vi "Insert Bundle Unbundle.vi"(8 "error in (no error)":errorcluster, 10 "Diagnostic VI Path":string, 11 "QD Launch VI Ref":refnum<vi>) -> (0 "error out":errorcluster, 3 "changes made?":bool)   [LabVIEW 2017]
doc: "把选中的多条 wire 按自上而下的位置顺序 Bundle 成一个 cluster，再 Unbundle 后接回原来的源端子与下游端子，数据流保持不变。\n\n限制：每根选中的 wire 只能有一个下游端子（无分叉）；有分叉时报错并放弃，不改动框图。\n\n输入：\nQD Launch VI Ref - QuickDrop 启动所在的 VI，取其 Block Diagram 的 Selection List[]（正常使用方式）。\nDiagnostic VI Path - 非空时改为打开该路径的 VI 并对该框图内所有 wire 操作，结束时保存该 VI（测试/批处理用）。\n\n输出：\nerror out - 选中对象不全是 wire、少于 2 根、或存在分叉时返回错误。\nchanges made? - 是否实际改动了框图。\n\nUndo 事务由调用方（QuickDrop 插件模板）管理。"
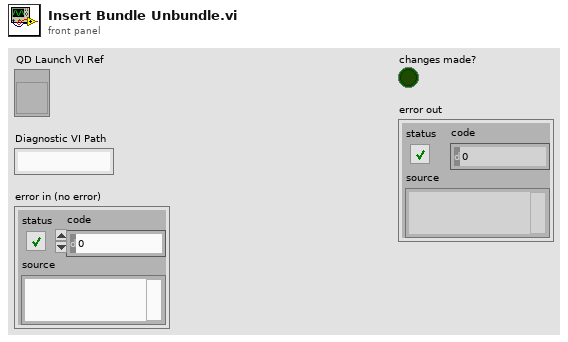
[diagram p1: front panel]
types:
  T1 = typedef "LVRectTypeDef.ctl" = cluster{"Left":i16, "Top":i16, "Right":i16, "Bottom":i16}
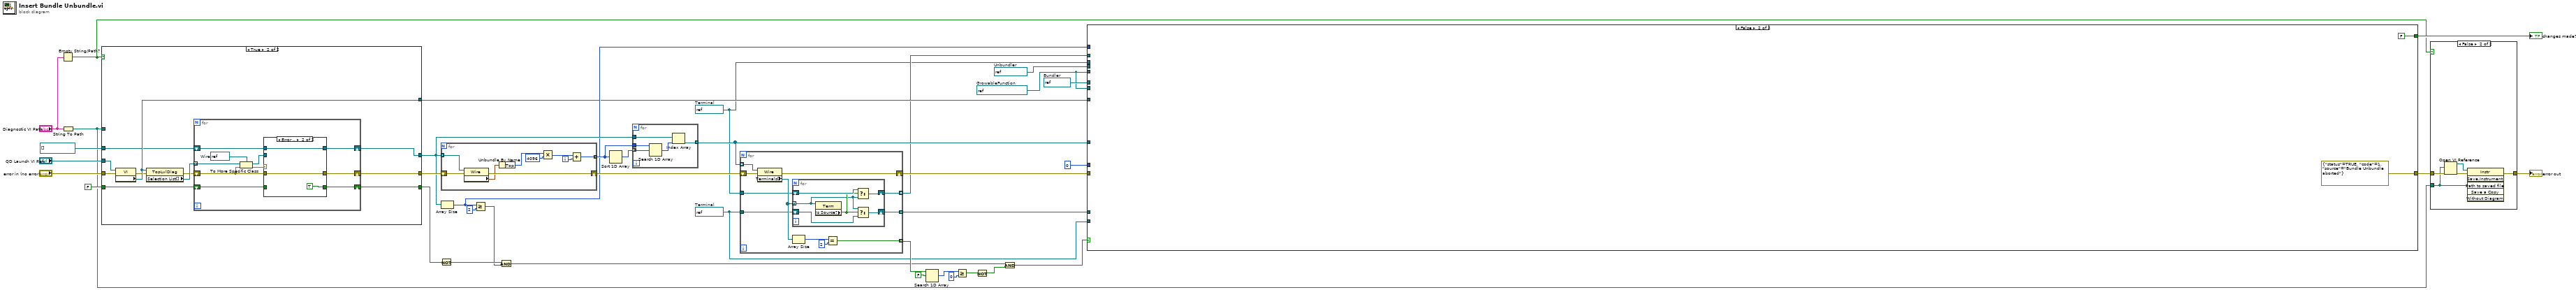
[diagram p0: block diagram]
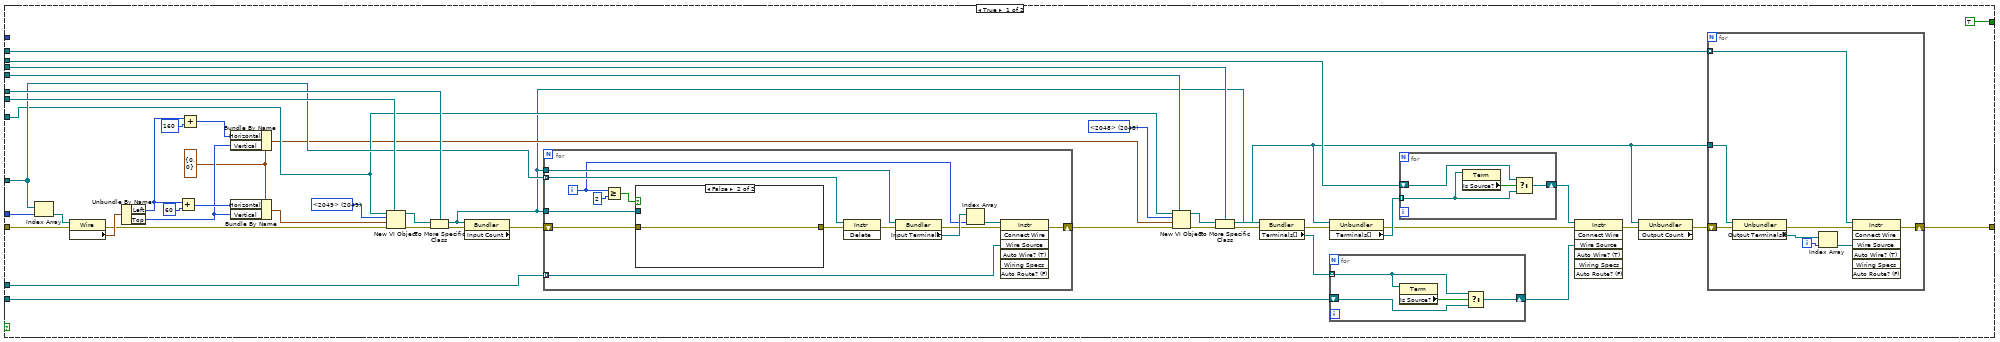
[diagram p3: hidden frame]
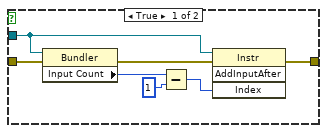
[diagram p4: hidden frame]
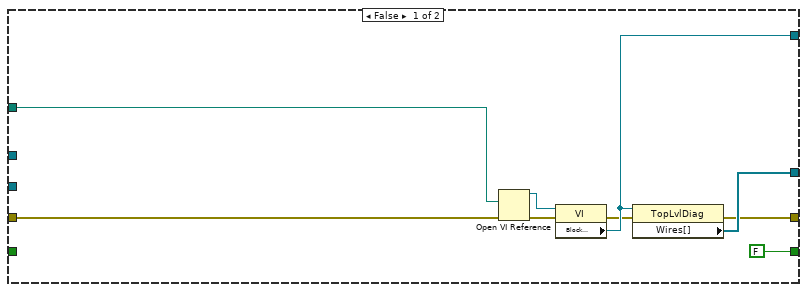
[diagram p5: hidden frame]
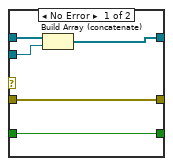
[diagram p6: hidden frame]
diagram:
  w7 = refnum<vi> refnum  # Terminal
  w8 = refnum<vi> refnum  # Terminal
  w10 = refnum<vi> refnum  # GrowableFunction
  w9 = refnum<vi> refnum  # Unbundler
  w11 = refnum<vi> refnum  # Bundler
  n1 = Empty String/Path?(string/path="Diagnostic VI Path") -> (empty?=w1:bool)
  n2 = String To Path(string="Diagnostic VI Path") -> (path=w4:path)
  n3 = case shown="True" w1 {
    tunnel: "error in (no error)" -> [w46 w58]
    tunnel: w4 -> [w47 _]
    tunnel: "QD Launch VI Ref" -> [_ w59]
    tunnel: [w40 w52] -> w34
    tunnel: [w41 w54] -> w25
    tunnel: [w43 w57] -> w15
    tunnel: [FALSE w50] -> w23
    tunnel: refnum<vi>[] [] -> [_ w53]
    tunnel: FALSE -> [_ w49]
    frame False {
      n4 = Open VI Reference(vi path=w47, error in (no error)=w46) -> (vi reference=w45:refnum<vi>, error out=w44:errorcluster)  [unwired: 4 in]
      n5 = property class="VI"(reference=w45, error in=w44) -> (error out=w42:errorcluster, "Block Diagram"=w43:refnum<vi>)  [unwired: 1 out]
      n6 = property class="TopLvlDiag"(reference=w43, error in=w42) -> (error out=w40:errorcluster, "Wires[]"=w41:refnum<vi>[])  [unwired: 1 out]
    }
    frame True {
      n7 = property class="VI"(reference=w59, error in=w58) -> (error out=w56:errorcluster, "Block Diagram"=w57:refnum<vi>)  [unwired: 1 out]
      n8 = property class="TopLvlDiag"(reference=w57, error in=w56) -> (error out=w51:errorcluster, "Selection List[]"=w55:refnum<vi>[])  [unwired: 1 out]
      n9 = for {
        tunnel: w55 -> [w69] mode=indexing
        shift-right: [w63] -> w54
        shift-left: w53 -> [w66]
        shift-right: [w61] -> w52
        shift-left: w51 -> [w67]
        shift-right: [w62] -> w50
        shift-left: w49 -> [w65]
        w68 = refnum<vi> refnum  # Wire
        n10 = To More Specific Class(target class=w68, reference=w69, error in=w67) -> (specific class reference=w64:refnum<vi>, error out=w60:errorcluster)
        n11 = case shown="Error .." w60 {
          tunnel: w67 -> [w73 w76]
          tunnel: w66 -> [w72 w77]
          tunnel: w65 -> [w74 _]
          tunnel: [w70 w77] -> w63
          tunnel: [w74 TRUE] -> w62
          tunnel: [w73 w76] -> w61
          tunnel: w64 -> [w71 _]
          frame No Error {
            n12 = Build Array (concatenate)(w72, w71) -> (w70:refnum<vi>[])
          }
          frame Error {
          }
        }
      }
    }
  }
  n13 = Not(x=w23) -> (.not. x?=w22:bool)
  n14 = for {
    tunnel: w25 -> [w86] mode=indexing
    tunnel: [w79] -> w32 mode=indexing
    shift-right: [w84] -> w31
    shift-left: w34 -> [w85]
    i -> [w78]
    n15 = property class="Wire"(reference=w86, error in=w85) -> (error out=w84:errorcluster, "Master Bounds Rect"=w83:T1)  [unwired: 1 out]
    n16 = Unbundle By Name(w83) -> ("Top"=w82:i16)
    n17 = Multiply(x=w82, y=4096) -> (x*y=w80:i32)
    n18 = Add(x=w80, y=w78) -> (x+y=w79:i32)
  }
  n19 = Array Size(array=w25) -> (size(s)=w16:i32)
  n20 = Greater Or Equal?(x=w16, y=2) -> (x >= y?=w21:bool)
  n21 = And(x=w22, y=w21) -> (x .and. y?=w20:bool)
  n22 = Sort 1D Array(array=w32) -> (sorted array=w33:i32[])
  n23 = for {
    tunnel: w33 -> [w90] mode=indexing
    tunnel: w32 -> [w91]
    tunnel: w25 -> [w89]
    tunnel: [w87] -> w17 mode=indexing
    n24 = Search 1D Array(1D array=w91, element=w90) -> (index of element=w88:i32)  [unwired: 1 in]
    n25 = Index Array(array=w89, index=w88) -> (element=w87:refnum<vi>)
  }
  n26 = for {
    tunnel: w17 -> [w102] mode=indexing
    shift-right: [w100] -> w18
    shift-left: w31 -> [w101]
    tunnel: [w97] -> w30 mode=indexing
    tunnel: [w95] -> w14 mode=indexing
    tunnel: [w93] -> w13 mode=indexing
    tunnel: w8 -> [w94]
    tunnel: w7 -> [w92]
    n27 = property class="Wire"(reference=w102, error in=w101) -> (error out=w100:errorcluster, "Terminals[]"=w96:refnum<vi>[])  [unwired: 1 out]
    n28 = for {
      tunnel: w96 -> [w104] mode=indexing
      shift-right: [w107] -> w95
      shift-left: w94 -> [w108]
      shift-right: [w103] -> w93
      shift-left: w92 -> [w106]
      n29 = property class="Term"(reference=w104) -> ("Is Source?"=w105:bool)  [unwired: 1 in, 2 out]
      n30 = Select(t=w106, s=w105, f=w104) -> (s? t:f=w103:refnum<vi>)
      n31 = Select(t=w104, s=w105, f=w108) -> (s? t:f=w107:refnum<vi>)
    }
    n32 = Array Size(array=w96) -> (size(s)=w99:i32)
    n33 = Equal?(x=w99, y=2) -> (x = y?=w97:bool)
  }
  n34 = Search 1D Array(1D array=w30, element=FALSE) -> (index of element=w28:i32)  [unwired: 1 in]
  n35 = Greater Or Equal?(x=w28, y=0) -> (x >= y?=w26:bool)
  n36 = Not(x=w26) -> (.not. x?=w19:bool)
  n37 = And(x=w20, y=w19) -> (x .and. y?=w5:bool)
  n38 = case shown="False" w5 {
    tunnel: w18 -> [w151 _]
    tunnel: w17 -> [w134 _]
    tunnel: w16 -> [_ _]
    tunnel: w15 -> [w131 _]
    tunnel: w14 -> [w133 _]
    tunnel: w13 -> [w112 _]
    tunnel: [w111 errorcluster {"status"=TRUE, "code"=1, "source"="Bundle Unbundle aborted"}] -> w3
    tunnel: [TRUE FALSE] -> w6
    tunnel: 0 -> [w153 _]
    tunnel: w10 -> [w139 _]
    tunnel: w11 -> [w136 _]
    tunnel: w10 -> [w127 _]
    tunnel: w9 -> [w124 _]
    tunnel: w8 -> [w120 _]
    tunnel: w7 -> [w117 _]
    frame True {
      w130 = 2048 items=[""=2041, "<2048>"=2048, "<2049>"=2049]
      w142 = 2049 items=[""=2041, "<2048>"=2048, "<2049>"=2049]
      w143 = cluster{"Horizontal":i16, "Vertical":i16} {"Horizontal"=0, "Vertical"=0}
      n39 = Index Array(array=w134, index=w153) -> (element=w152:refnum<vi>)
      n40 = property class="Wire"(reference=w152, error in=w151) -> (error out=w140:errorcluster, "Master Bounds Rect"=w150:T1)  [unwired: 1 out]
      n41 = Unbundle By Name(w150) -> ("Left"=w148:i16, "Top"=w144:i16)
      n42 = Add(x=w148, y=60) -> (x+y=w146:i32)
      n43 = Add(x=w148, y=160) -> (x+y=w145:i32)
      n44 = Bundle By Name(cluster=w143, "Horizontal"=w145, "Vertical"=w144) -> (w129:cluster{"Horizontal":i16, "Vertical":i16})
      n45 = Bundle By Name(cluster=w143, "Horizontal"=w146, "Vertical"=w144) -> (w141:cluster{"Horizontal":i16, "Vertical":i16})
      n46 = New VI Object(vi object class=w139, owner refnum=w131, style=w142, position/next to=w141, 8:w140) -> (object refnum=w138:refnum<vi>, 0:w137:errorcluster)  [unwired: 3 in]
      n47 = To More Specific Class(target class=w136, reference=w138, error in=w137) -> (specific class reference=w123:refnum<vi>, error out=w135:errorcluster)
      n48 = property class="Bundler" props=["Input Count"](reference=w123, error in=w135) -> (error out=w132:errorcluster)  [unwired: 2 out]
      n49 = for {
        tunnel: w134 -> [w180] mode=indexing
        tunnel: w133 -> [w173] mode=indexing
        shift-right: [w172] -> w128
        shift-left: w132 -> [w183]
        tunnel: w123 -> [w182]
        tunnel: w123 -> [w178]
        i -> [w171]
        n50 = Greater Or Equal?(x=w171, y=2) -> (x >= y?=w181:bool)
        n51 = case shown="False" w181 {
          tunnel: w183 -> [w191 w192]
          tunnel: w182 -> [w188 _]
          tunnel: [w185 w192] -> w179
          frame True {
            n52 = property class="Bundler"(reference=w188, error in=w191) -> (error out=w187:errorcluster, "Input Count"=w190:i32)  [unwired: 1 out]
            n53 = Subtract(x=w190, y=1) -> (x-y=w186:i32)
            n54 = invoke class="Instr" method="AddInputAfter"(reference=w188, error in=w187, "Index"=w186) -> (error out=w185:errorcluster)  [unwired: 1 in, 3 out]
          }
          frame False {
          }
        }
        n55 = invoke class="Instr" method="Delete"(reference=w180, error in=w179) -> (error out=w177:errorcluster)  [unwired: 1 in, 2 out]
        n56 = property class="Bundler"(reference=w178, error in=w177) -> (error out=w174:errorcluster, "Input Terminals"=w176:refnum<vi>[])  [unwired: 1 out]
        n57 = Index Array(array=w176, index=w171) -> (element=w175:refnum<vi>)
        n58 = invoke class="Instr" method="Connect Wire"(reference=w175, error in=w174, "Wire Source"=w173) -> (error out=w172:errorcluster)  [unwired: 4 in, 6 out]
      }
      n59 = New VI Object(vi object class=w127, owner refnum=w131, style=w130, position/next to=w129, 8:w128) -> (object refnum=w126:refnum<vi>, 0:w125:errorcluster)  [unwired: 3 in]
      n60 = To More Specific Class(target class=w124, reference=w126, error in=w125) -> (specific class reference=w109:refnum<vi>, error out=w122:errorcluster)
      n61 = property class="Bundler"(reference=w123, error in=w122) -> (error out=w119:errorcluster, "Terminals[]"=w121:refnum<vi>[])  [unwired: 1 out]
      n62 = property class="Unbundler"(reference=w109, error in=w119) -> (error out=w115:errorcluster, "Terminals[]"=w118:refnum<vi>[])  [unwired: 1 out]
      n63 = for {
        tunnel: w121 -> [w170] mode=indexing
        shift-right: [w167] -> w114
        shift-left: w120 -> [w168]
        n64 = property class="Term"(reference=w170) -> ("Is Source?"=w169:bool)  [unwired: 1 in, 2 out]
        n65 = Select(t=w170, s=w169, f=w168) -> (s? t:f=w167:refnum<vi>)
      }
      n66 = for {
        tunnel: w118 -> [w164] mode=indexing
        shift-right: [w163] -> w116
        shift-left: w117 -> [w166]
        n67 = property class="Term"(reference=w164) -> ("Is Source?"=w165:bool)  [unwired: 1 in, 2 out]
        n68 = Select(t=w166, s=w165, f=w164) -> (s? t:f=w163:refnum<vi>)
      }
      n69 = invoke class="Instr" method="Connect Wire"(reference=w116, error in=w115, "Wire Source"=w114) -> (error out=w113:errorcluster)  [unwired: 4 in, 6 out]
      n70 = property class="Unbundler" props=["Output Count"](reference=w109, error in=w113) -> (error out=w110:errorcluster)  [unwired: 2 out]
      n71 = for {
        tunnel: w112 -> [w159] mode=indexing
        shift-right: [w156] -> w111
        shift-left: w110 -> [w161]
        tunnel: w109 -> [w162]
        i -> [w155]
        n72 = property class="Unbundler"(reference=w162, error in=w161) -> (error out=w158:errorcluster, "Output Terminals[]"=w160:refnum<vi>[])  [unwired: 1 out]
        n73 = Index Array(array=w160, index=w155) -> (element=w157:refnum<vi>)
        n74 = invoke class="Instr" method="Connect Wire"(reference=w159, error in=w158, "Wire Source"=w157) -> (error out=w156:errorcluster)  [unwired: 4 in, 6 out]
      }
    }
    frame False {
    }
  }
  "changes made?" <- w6
  n75 = case shown="False" w1 {
    tunnel: w4 -> [_ w197]
    tunnel: w3 -> [w195 w200]
    tunnel: [w195 w196] -> w2
    frame True {
    }
    frame False {
      n76 = Open VI Reference(vi path=w197, error in (no error)=w200) -> (vi reference=w199:refnum<vi>, error out=w198:errorcluster)  [unwired: 4 in]
      n77 = invoke class="Instr" method="Save.Instrument"(reference=w199, error in=w198, "Path to saved file"=w197) -> (error out=w196:errorcluster)  [unwired: 3 in, 5 out]
    }
  }
  "error out" <- w2
